vi "PNA_Sparameter_field_sweep.vi"() -> ()   [LabVIEW 2015]
uses:
  <vilib>/Utility/file.llb/Write To Spreadsheet File (string).vi
panel:
  out "Field Point":i32
  in  "Averages":i32
  out "Field (Oe)":dbl
  in  "Beep when done":bool
  out "XY Graph":cluster{dbl[], "Array":dbl[]}(graph)
  in  "VNA":refnum<visa-resource-name>="GPIB0::16::INSTR"
  in  "File Note (Optional)":string
  in  "Response Cal":bool
  in  "Format":string(combo)="MLOG"
  in  "Measurement":string(combo)="S21"
  in  "VNA Number of Points":string="1601"
  in  "Save location":path=path "C:/Users/probe_station/Desktop/VNA Data"
  in  "Field Points":dbl=21.0
  in  "Field Stop (A)":dbl=3.0
  in  "Field Start (A)":dbl=-3.0
  in  "Frequency Stop (GHz)":dbl=4.0
  in  "Frequency Start (GHz)":dbl=1.0
  in  "Gaussmeter GPIB Address":string="22"
  in  "Power Supply GPIB Address":string="6"
  in  "VNA GPIB Address":string="16"
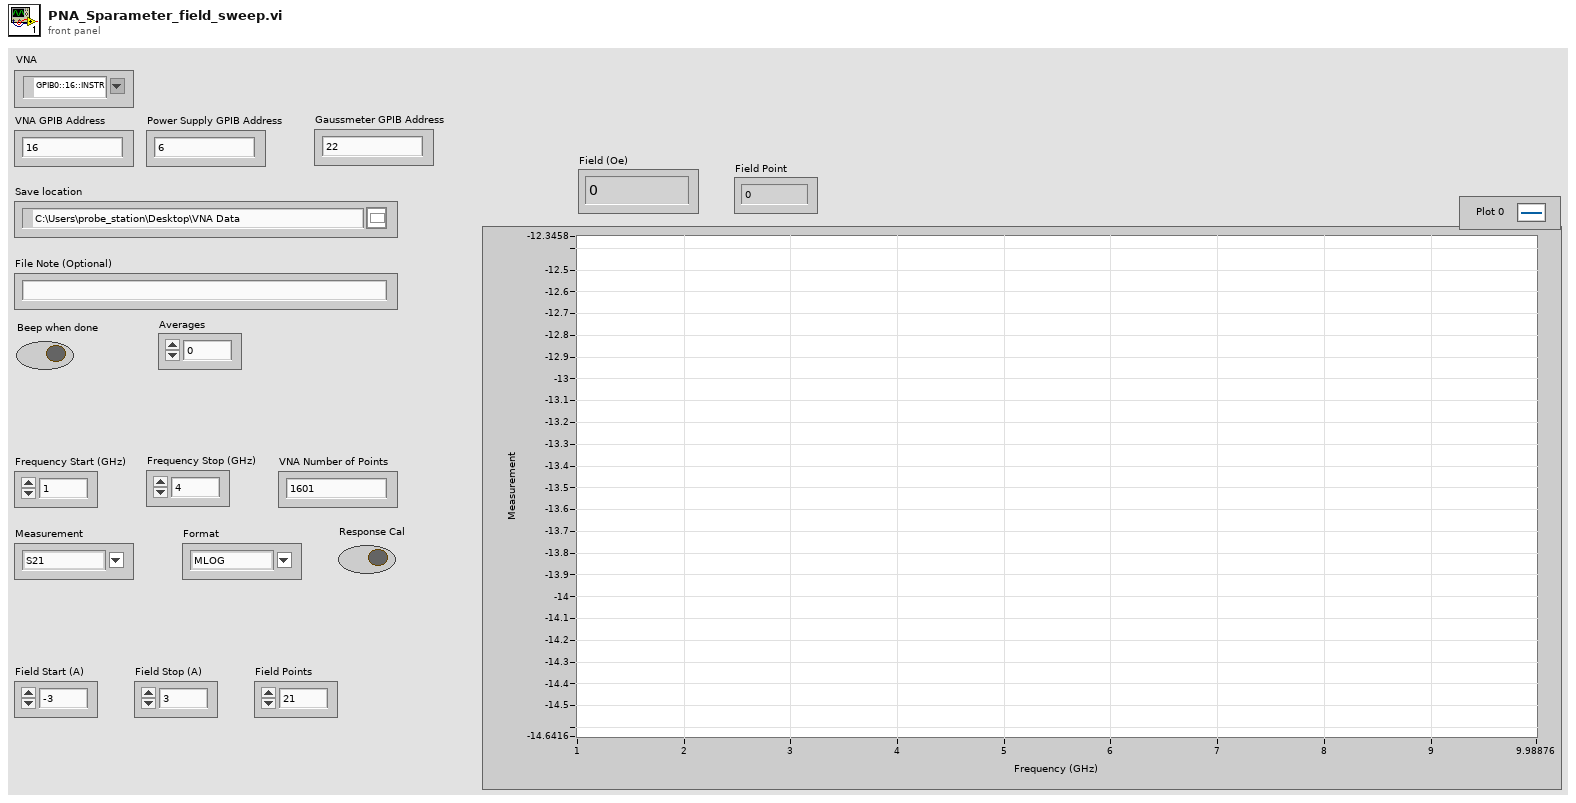
[diagram p1: front panel]
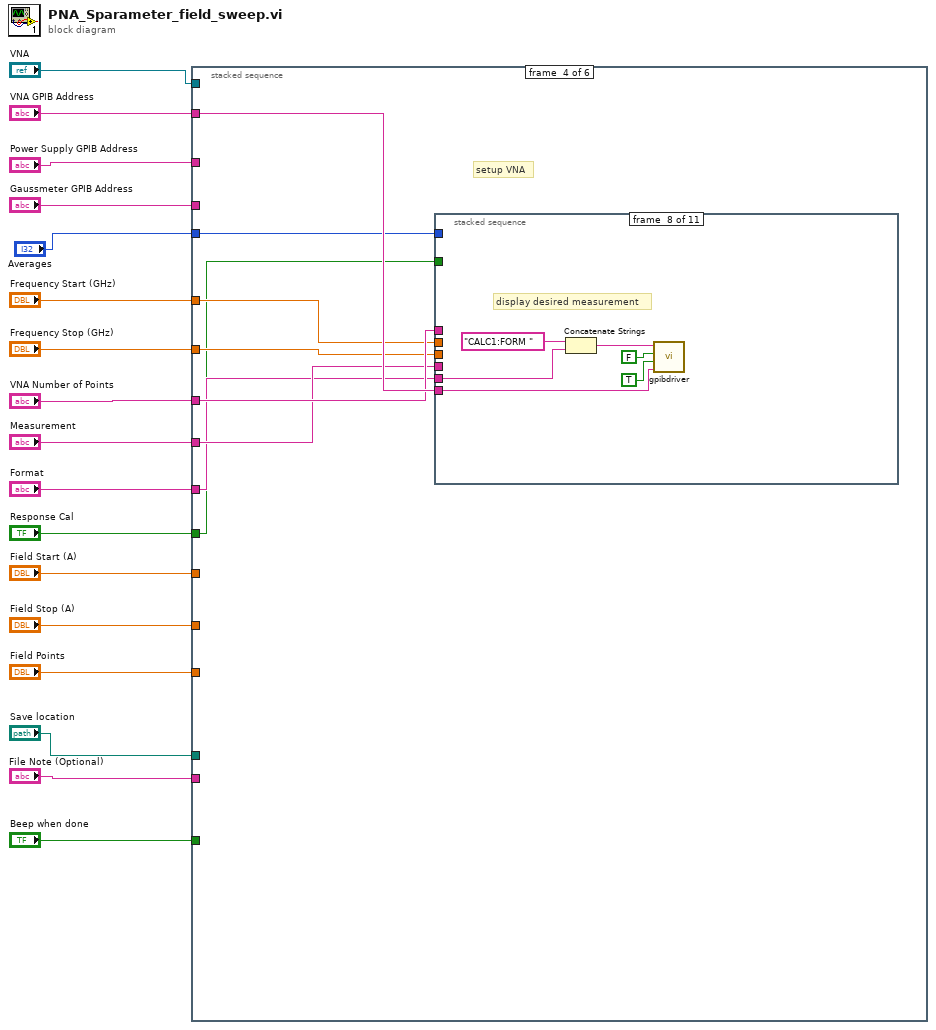
[diagram p0: block diagram]
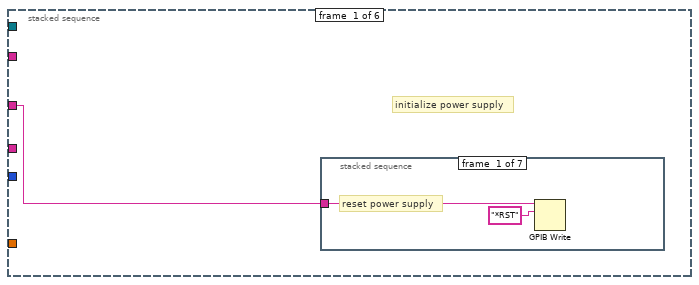
[diagram p2: hidden frame]
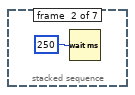
[diagram p3: hidden frame]
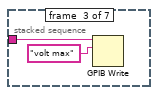
[diagram p4: hidden frame]
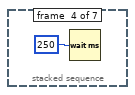
[diagram p5: hidden frame]
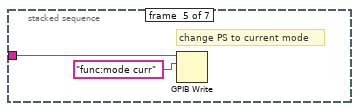
[diagram p6: hidden frame]
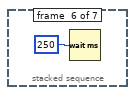
[diagram p7: hidden frame]
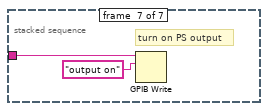
[diagram p8: hidden frame]
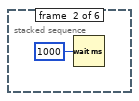
[diagram p9: hidden frame]
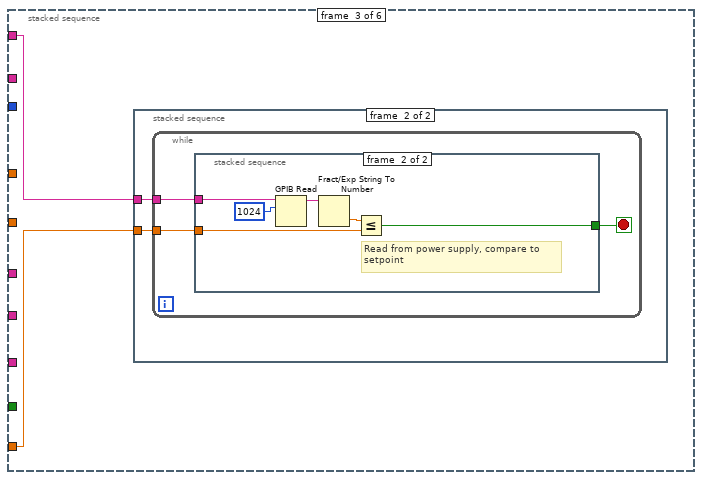
[diagram p10: hidden frame]
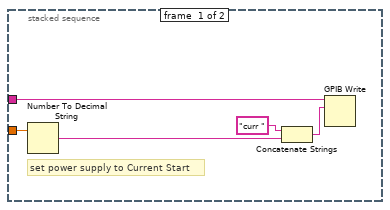
[diagram p11: hidden frame]
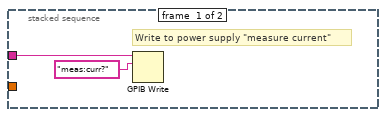
[diagram p12: hidden frame]
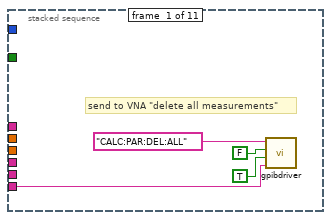
[diagram p13: hidden frame]
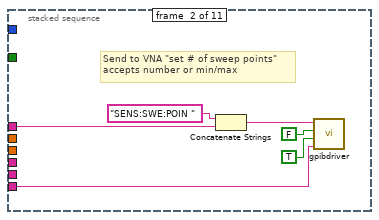
[diagram p14: hidden frame]
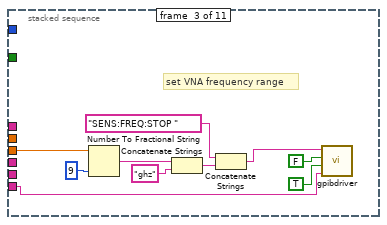
[diagram p15: hidden frame]
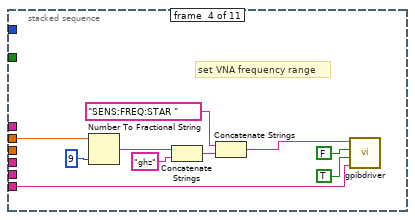
[diagram p16: hidden frame]
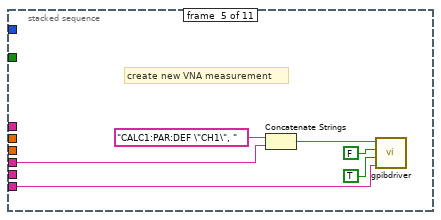
[diagram p17: hidden frame]
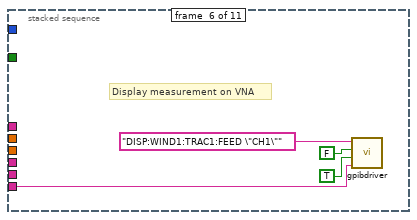
[diagram p18: hidden frame]
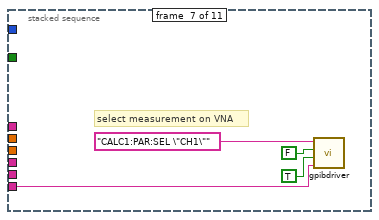
[diagram p19: hidden frame]
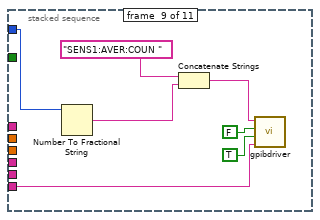
[diagram p20: hidden frame]
diagram:
  n1 = stacked-sequence {
    tunnel: "Power Supply GPIB Address" -> [w18 _ w32 _ w162 w266]
    tunnel: "Field Start (A)" -> [_ _ w31 _ w161 _]
    tunnel: "VNA GPIB Address" -> [_ _ _ w58 w159 _]
    tunnel: "VNA Number of Points" -> [_ _ _ w57 w157 _]
    tunnel: "Frequency Start (GHz)" -> [_ _ _ w56 w155 _]
    tunnel: "Frequency Stop (GHz)" -> [_ _ _ w55 w156 _]
    tunnel: "Measurement" -> [_ _ _ w54 w150 _]
    tunnel: "Format" -> [_ _ _ w53 w149 _]
    tunnel: "Response Cal" -> [_ _ _ w52 _ _]
    tunnel: "Field Points" -> [_ _ _ _ w163 _]
    tunnel: "Field Stop (A)" -> [_ _ _ _ w160 _]
    tunnel: "VNA" -> [_ _ _ _ w158 _]
    tunnel: "Save location" -> [_ _ _ _ w152 _]
    tunnel: "File Note (Optional)" -> [_ _ _ _ w151 _]
    tunnel: "Gaussmeter GPIB Address" -> [_ _ _ _ w148 _]
    tunnel: "Beep when done" -> [_ _ _ _ _ w264]
    tunnel: "Averages" -> [_ _ _ w51 w147 _]
    frame #0 {
      # "initialize power supply"
      n2 = stacked-sequence {
        tunnel: w18 -> [w19 _ w23 _ w26 _ w29]
        frame #0 {
          # "reset power supply"
          n3 = GPIB Write(0:w19, 1:"*RST" ("data")) -> ()  [unwired: 3 in, 2 out]
        }
        frame #1 {
          n4 = Wait (ms)(milliseconds to wait=u32 250) -> ()  [unwired: 1 out]
        }
        frame #2 {
          n5 = GPIB Write(0:w23, 1:"volt max" ("data")) -> ()  [unwired: 3 in, 2 out]
        }
        frame #3 {
          n6 = Wait (ms)(milliseconds to wait=u32 250) -> ()  [unwired: 1 out]
        }
        frame #4 {
          # "change PS to current mode"
          n7 = GPIB Write(0:w26, 1:"func:mode curr" ("data")) -> ()  [unwired: 3 in, 2 out]
        }
        frame #5 {
          n8 = Wait (ms)(milliseconds to wait=u32 250) -> ()  [unwired: 1 out]
        }
        frame #6 {
          # "turn on PS output"
          n9 = GPIB Write(0:w29, 1:"output on" ("data")) -> ()  [unwired: 3 in, 2 out]
        }
      }
    }
    frame #1 {
      n10 = Wait (ms)(milliseconds to wait=u32 1000) -> ()  [unwired: 1 out]
    }
    frame #2 {
      n11 = stacked-sequence {
        tunnel: w32 -> [w37 w39]
        tunnel: w31 -> [w34 w38]
        frame #0 {
          # "set power supply to Current Start"
          n12 = Number To Decimal String(number=w34) -> (decimal integer string=w33:string)  [unwired: 1 in]
          n13 = Concatenate Strings("curr " ("string"), w33) -> (w35:string)
          n14 = GPIB Write(0:w37, 1:w35) -> ()  [unwired: 3 in, 2 out]
        }
        frame #1 {
          n15 = while {
            tunnel: w39 -> [w41]
            tunnel: w38 -> [w40]
            stop <- w42 stop-if-true
            n16 = stacked-sequence {
              tunnel: [_ w50] -> w42
              tunnel: w41 -> [w44 w48]
              tunnel: w40 -> [_ w49]
              frame #0 {
                # "Write to power supply \"measure current\""
                n17 = GPIB Write(0:w44, 1:"meas:curr?" ("data")) -> ()  [unwired: 3 in, 2 out]
              }
              frame #1 {
                # "Read from power supply, compare to\nsetpoint"
                n18 = GPIB Read(0:w48, 1:1024 ("byte count")) -> (5:w47:string)  [unwired: 3 in, 2 out]
                n19 = Fract/Exp String To Number(string=w47) -> (number=w46:dbl)  [unwired: 3 in, 1 out]
                n20 = Less Or Equal?(x=w46, y=w49) -> (x <= y?=w50:bool)
              }
            }
          }
        }
      }
    }
    frame #3 {
      # "setup VNA"
      n21 = stacked-sequence {
        tunnel: w58 -> [w59 w64 w74 w84 w92 w95 w99 w103 w113 w116 w143]
        tunnel: w57 -> [_ w63 _ _ _ _ _ _ _ _ _]
        tunnel: w56 -> [_ _ _ w80 _ _ _ _ _ _ _]
        tunnel: w55 -> [_ _ w73 _ _ _ _ _ _ _ _]
        tunnel: w54 -> [_ _ _ _ w89 _ _ _ _ _ _]
        tunnel: w53 -> [_ _ _ _ _ _ _ w104 _ _ _]
        tunnel: w52 -> [_ _ _ _ _ _ _ _ _ w117 _]
        tunnel: w51 -> [_ _ _ _ _ _ _ _ w112 _ _]
        frame #0 {
          # "send to VNA \"delete all measurements\""
          n22 = call "gpibdriver.vi"("Characters to Write"="CALC:PAR:DEL:ALL", "Read"=FALSE, "Write"=TRUE ("Write 3"), "GPIB\nAddress"=w59) -> ()  [unwired: 2 in, 1 out]
        }
        frame #1 {
          # "Send to VNA \"set # of sweep points\"\naccepts number or min/max"
          n23 = Concatenate Strings("SENS:SWE:POIN " ("Characters to Write"), w63) -> (w68:string)
          n24 = call "gpibdriver.vi"("Characters to Write"=w68, "Read"=FALSE, "Write"=TRUE, "GPIB\nAddress"=w64) -> ()  [unwired: 2 in, 1 out]
        }
        frame #2 {
          # "set VNA frequency range"
          n25 = Number To Fractional String(number=w73, precision (6)=i16 9) -> (F-format string=w71:string)  [unwired: 2 in]
          n26 = Concatenate Strings(w71, "ghz" ("string")) -> (w69:string)
          n27 = Concatenate Strings("SENS:FREQ:STOP " ("Characters to Write"), w69) -> (w77:string)
          n28 = call "gpibdriver.vi"("Characters to Write"=w77, "Read"=FALSE, "Write"=TRUE ("Write 3"), "GPIB\nAddress"=w74) -> ()  [unwired: 2 in, 1 out]
        }
        frame #3 {
          # "set VNA frequency range"
          n29 = Number To Fractional String(number=w80, precision (6)=i16 9) -> (F-format string=w82:string)  [unwired: 2 in]
          n30 = Concatenate Strings(w82, "ghz" ("string")) -> (w79:string)
          n31 = Concatenate Strings("SENS:FREQ:STAR " ("Characters to Write"), w79) -> (w87:string)
          n32 = call "gpibdriver.vi"("Characters to Write"=w87, "Read"=FALSE, "Write"=TRUE ("Write 3"), "GPIB\nAddress"=w84) -> ()  [unwired: 2 in, 1 out]
        }
        frame #4 {
          # "create new VNA measurement"
          n33 = Concatenate Strings("CALC1:PAR:DEF \"CH1\", " ("Characters to Write"), w89) -> (w90:string)
          n34 = call "gpibdriver.vi"("Characters to Write"=w90, "Read"=FALSE, "Write"=TRUE ("Write 3"), "GPIB\nAddress"=w92) -> ()  [unwired: 2 in, 1 out]
        }
        frame #5 {
          # "Display measurement on VNA"
          n35 = call "gpibdriver.vi"("Characters to Write"="DISP:WIND1:TRAC1:FEED \"CH1\"", "Read"=FALSE, "Write"=TRUE ("Write 3"), "GPIB\nAddress"=w95) -> ()  [unwired: 2 in, 1 out]
        }
        frame #6 {
          # "select measurement on VNA"
          n36 = call "gpibdriver.vi"("Characters to Write"="CALC1:PAR:SEL \"CH1\"", "Read"=FALSE, "Write"=TRUE ("Write 3"), "GPIB\nAddress"=w99) -> ()  [unwired: 2 in, 1 out]
        }
        frame #7 {
          # "display desired measurement"
          n37 = Concatenate Strings("CALC1:FORM " ("Characters to Write"), w104) -> (w105:string)
          n38 = call "gpibdriver.vi"("Characters to Write"=w105, "Read"=FALSE, "Write"=TRUE ("Write 3"), "GPIB\nAddress"=w103) -> ()  [unwired: 2 in, 1 out]
        }
        frame #8 {
          n39 = Number To Fractional String(number=w112) -> (F-format string=w111:string)  [unwired: 3 in]
          n40 = Concatenate Strings("SENS1:AVER:COUN " ("string"), w111) -> (w109:string)
          n41 = call "gpibdriver.vi"("Characters to Write"=w109, "Read"=FALSE, "Write"=TRUE ("Write 3"), "GPIB\nAddress"=w113) -> ()  [unwired: 2 in, 1 out]
        }
        frame #9 {
          # "Response Cal?"
          n42 = case shown="True" w117 {
            tunnel: w116 -> [_ w118]
            frame False {
            }
            frame True {
              n43 = stacked-sequence {
                tunnel: w118 -> [w119 w123 w127 w131 w135 w139]
                frame #0 {
                  # "set ch 1 calibratoin to Response Thru"
                  n44 = call "gpibdriver.vi"("Characters to Write"="SENS:CORR:COLL:METH TRAN1", "Read"=FALSE, "Write"=TRUE, "GPIB\nAddress"=w119) -> ()  [unwired: 2 in, 1 out]
                }
                frame #1 {
                  # "operation complete?"
                  n45 = call "gpibdriver.vi"("Characters to Write"="*OPC?", "Read"=TRUE, "Write"=TRUE ("Write 2"), "GPIB\nAddress"=w123) -> ()  [unwired: 2 in, 1 out]
                }
                frame #2 {
                  # "measure the calibration standard\n(not 100% sure on this one)"
                  n46 = call "gpibdriver.vi"("Characters to Write"="SENS:CORR:COLL STAN4", "Read"=FALSE, "Write"=TRUE, "GPIB\nAddress"=w127) -> ()  [unwired: 2 in, 1 out]
                }
                frame #3 {
                  # "operation complete?"
                  n47 = call "gpibdriver.vi"("Characters to Write"="*OPC?", "Read"=TRUE, "Write"=TRUE ("Write 2"), "GPIB\nAddress"=w131) -> ()  [unwired: 2 in, 1 out]
                }
                frame #4 {
                  # "save calibration"
                  n48 = call "gpibdriver.vi"("Characters to Write"="SENS:CORR:COLL:SAVE", "Read"=FALSE, "Write"=TRUE, "GPIB\nAddress"=w135) -> ()  [unwired: 2 in, 1 out]
                }
                frame #5 {
                  # "operation complete?"
                  n49 = call "gpibdriver.vi"("Characters to Write"="*OPC?", "Read"=TRUE, "Write"=TRUE ("Write 2"), "GPIB\nAddress"=w139) -> ()  [unwired: 2 in, 1 out]
                }
              }
            }
          }
        }
        frame #10 {
          # "set manual sweep on VNA"
          n50 = call "gpibdriver.vi"("Characters to Write"="INIT:CONT OFF", "Read"=FALSE, "Write"=TRUE, "GPIB\nAddress"=w143) -> ()  [unwired: 2 in, 1 out]
        }
      }
    }
    frame #4 {
      # "Create frequency array"
      n51 = Fract/Exp String To Number(string=w157) -> (number=w153:dbl)  [unwired: 3 in, 1 out]
      n52 = for {
        N: w153 -> [w174]
        tunnel: w156 -> [w175]
        tunnel: w155 -> [w167]
        shift-right: [w165] -> w154
        shift-left: _ -> [w164]
        i -> [w170]
        n53 = Subtract(x=w175, y=w167) -> (x-y=w172:dbl)
        n54 = Add(x=w174, y=1) -> (x+y=w171:i32)
        n55 = Divide(x=w172, y=w171) -> (x/y=w169:dbl)
        n56 = Multiply(x=w169, y=w170) -> (x*y=w168:dbl)
        n57 = Add(x=w168, y=w167) -> (x+y=w166:dbl)
        n58 = Build Array (concatenate)(w166, w164) -> (w165:dbl[])
      }
      n59 = for {
        N: w163 -> [w190]
        tunnel: w162 -> [w189]
        tunnel: w161 -> [w188]
        tunnel: w160 -> [w187]
        tunnel: w159 -> [w186]
        tunnel: w158 -> [w185]
        tunnel: w157 -> [w184]
        tunnel: w154 -> [w183]
        tunnel: w152 -> [w182]
        tunnel: w151 -> [w181]
        tunnel: w150 -> [w180]
        tunnel: w149 -> [w179]
        tunnel: w148 -> [w178]
        tunnel: w147 -> [w177]
        i -> [w176]
        n60 = stacked-sequence {
          seq-local: [w191 _ _ _ _ _] -> [_ _ _ _ _ w225]
          tunnel: w187 -> [w203 _ _ _ _ _]
          tunnel: w188 -> [w198 _ _ _ _ _]
          tunnel: w190 -> [w193 _ _ _ _ _]
          tunnel: w176 -> [w201 _ _ _ _ _]
          tunnel: w189 -> [w194 _ _ _ _ _]
          tunnel: w186 -> [_ _ w206 w216 _ _]
          tunnel: w185 -> [_ _ _ _ _ w259]
          tunnel: w184 -> [_ _ _ _ _ _]
          tunnel: w183 -> [_ _ _ _ _ w222]
          tunnel: w182 -> [_ _ _ _ _ w251]
          tunnel: w181 -> [_ _ _ _ _ w229]
          tunnel: w180 -> [_ _ _ _ _ w240]
          tunnel: w179 -> [_ _ _ _ _ w237]
          tunnel: w178 -> [_ _ _ _ _ w232]
          tunnel: w177 -> [_ _ w205 _ _ _]
          frame #0 {
            # "set power supply current"
            n61 = Subtract(x=w203, y=w198) -> (x-y=w202:dbl)
            n62 = Divide(x=w202, y=w193) -> (x/y=w200:dbl)
            n63 = Multiply(x=w200, y=w201) -> (x*y=w199:dbl)
            n64 = Add(x=w199, y=w198) -> (x+y=w192:dbl)
            n65 = Less Than 0?(x=w192) -> (x < 0?=w191:bool)
            n66 = Number To Fractional String(number=w192) -> (F-format string=w195:string)  [unwired: 3 in]
            n67 = Concatenate Strings("curr " ("string"), w195) -> (w197:string)
            n68 = GPIB Write(0:w194, 1:w197) -> ()  [unwired: 3 in, 2 out]
          }
          frame #1 {
            n69 = Wait (ms)(milliseconds to wait=u32 1000) -> ()  [unwired: 1 out]
          }
          frame #2 {
            # "Trigger VNA measurement"
            n70 = for {
              N: w205 -> [_]
              tunnel: w206 -> [w207]
              n71 = stacked-sequence {
                tunnel: w207 -> [w208 w212]
                frame #0 {
                  n72 = call "gpibdriver.vi"("Characters to Write"="INIT", "Read"=FALSE, "Write"=TRUE ("Write 2"), "GPIB\nAddress"=w208) -> ()  [unwired: 2 in, 1 out]
                }
                frame #1 {
                  # "operation complete?"
                  n73 = call "gpibdriver.vi"("Characters to Write"="*OPC?", "Read"=TRUE, "Write"=TRUE ("Write 2"), "GPIB\nAddress"=w212) -> ()  [unwired: 2 in, 1 out]
                }
              }
            }
          }
          frame #3 {
            # "Select channel 1 measurement"
            n74 = call "gpibdriver.vi"("Characters to Write"="CALC1:PAR:SEL \"CH1\"", "Read"=FALSE, "Write"=TRUE ("Write 2"), "GPIB\nAddress"=w216) -> ()  [unwired: 2 in, 1 out]
          }
          frame #4 {
            n75 = Wait (ms)(milliseconds to wait=u32 2000) -> ()  [unwired: 1 out]
          }
          frame #5 {
            # "Write output"
            # "add date/time & H field to file name"
            # "Read H field"
            # "Read measurement"
            n76 = Reverse 1D Array(array=w222) -> (reversed array=w221:dbl[])
            n77 = call "VNA read data new.vi"("Data Type"="FDATA", "Channel"=1.0, "VISA resource name"=w259) -> ("Array"=w258:dbl[])  [unwired: 1 in]
            n78 = call "Field_from_HP3478A.vi"("GPIB Address"=w232) -> ("Oe"=w233:dbl)  [unwired: 2 out]
            "Field (Oe)" <- w233
            n79 = Number To Fractional String(number=w258) -> (F-format string=w224:string[])  [unwired: 3 in]
            n80 = Number To Fractional String(number=w221) -> (F-format string=w245:string[])  [unwired: 3 in]
            n81 = Get Date/Time In Seconds() -> (seconds since 1Jan1904=w249:timestamp)
            n82 = Bundle(w221, "Array"=w258) -> (→"XY Graph":cluster{dbl[], "Array":dbl[]})  [unwired: 1 in]
            n83 = case shown="True" w225 {
              tunnel: ["+" ("string") "-" ("string")] -> w226
              frame False {
              }
              frame True {
              }
            }
            n84 = Reverse 1D Array(array=w224) -> (reversed array=w223:string[])
            n85 = Concatenate Strings(w240, " (" ("string"), w237, ")" ("string")) -> (w236:string)
            n86 = Reverse 1D Array(array=w245) -> (reversed array=w244:string[])
            n87 = Format Date/Time String(time format string (%c)="%Y_%m_%d_%H_%M_%S;", seconds (now)=w249) -> (date/time string=w247:string)  [unwired: 1 in]
            n88 = Number To Fractional String(number=w233, precision (6)=i16 2) -> (F-format string=w227:string)  [unwired: 2 in]
            n89 = Build Array (concatenate)(w223, w236) -> (w235:string[])
            n90 = Build Array (concatenate)(w244, "Frequency (GHz)" ("time format string (%c)")) -> (w242:string[])
            n91 = Reverse 1D Array(array=w235) -> (reversed array=w234:string[])
            n92 = Reverse 1D Array(array=w242) -> (reversed array=w241:string[])
            n93 = Concatenate Strings(w247, w226, w227, "Oe_" ("string"), w229, ".txt" ("string")) -> (w246:string)
            n94 = Build Array(w241, w234) -> (w256:string[][])
            n95 = Path To String(path=w251) -> (string=w254:string)
            n96 = Transpose 2D Array(2D array=w256) -> (transposed array=w255:string[][])
            n97 = Concatenate Strings(w254, "\\" ("string"), w246) -> (w252:string)
            n98 = String To Path(string=w252) -> (path=w250:path)
            n99 = call-poly <vilib>:"Write To Spreadsheet File.vi"("2D data"=w255, "file path (dialog if empty)"=w250) -> ()  [unwired: 6 in, 1 out]
          }
        }
        "Field Point" <- w176
      }
    }
    frame #5 {
      # "Reset power supply"
      n100 = case shown="True" w264 {
        tunnel: ["*RST" ("data") "*RST;syst:beep" ("data")] -> w265
        frame False {
        }
        frame True {
        }
      }
      n101 = GPIB Write(0:w266, 1:w265) -> ()  [unwired: 3 in, 2 out]
    }
  }
